vi "IR - Volt to cm.vi"(5 "Volt":u16) -> (2 "Distance (cm)":dbl)   [LabVIEW 2019]
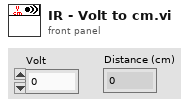
[diagram p1: front panel]
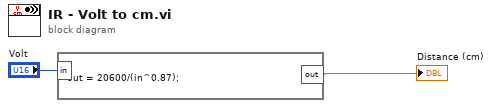
[diagram p0: block diagram]
diagram:
  n1 = formula code="out = 20600/(in^0.87);"("in"="Volt") -> ("out"=→"Distance (cm)":dbl)
